vi "Test Type Check L2.vi"() -> ()   [LabVIEW 2021]
uses:
  ChannelCommon/typedef/FIFO Config.ctl
  ChannelCommon/ChannelCommon.lvlib
  CIFChannels/Typedef/Direction.ctl
  CIFChannels/CIFChannels.lvclass
  ChannelCommon/typedef/TimeStamps.ctl
  CIF_CIPC_L2Enet.lvclass
  FIFO_U8/CIF_CIPC_Fifo_U8.lvclass
  FIFO_Universal/CIF_CIPC_Universal.lvclass
panel:
  out "status":string
  out "pass":bool
  out "error out":errorcluster
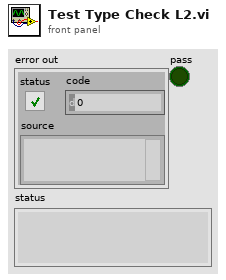
[diagram p1: front panel]
types:
  T1 = typedef "CIFChannels.lvclass/Direction.ctl" = enum16{"Publisher", "Subscriber"}
  T2 = typedef "ChannelCommon.lvlib/TimeStamps.ctl" = cluster{"ClockID":u8, "T0":i64, "T_Out":i64}
  T3 = typedef "ChannelCommon.lvlib/FIFO Config.ctl" = cluster{"Max Bytes/Msg":u64, "Max Msg/FIFO":u64, "Flags":u64}
  T4 = typedef "ChannelCommon.lvlib/New FIFO Instance Response.ctl" = cluster{"Publisher":string, "Custom Data":u8[]}
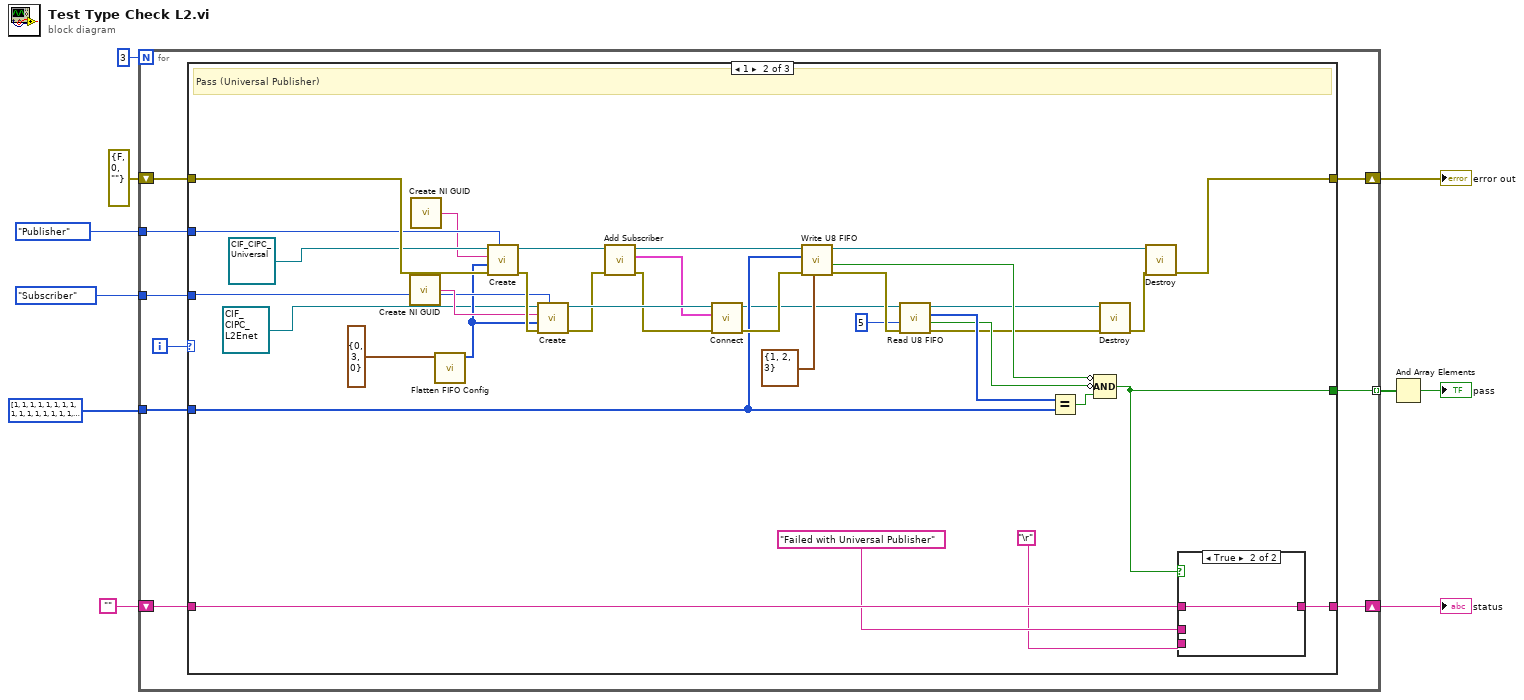
[diagram p0: block diagram]
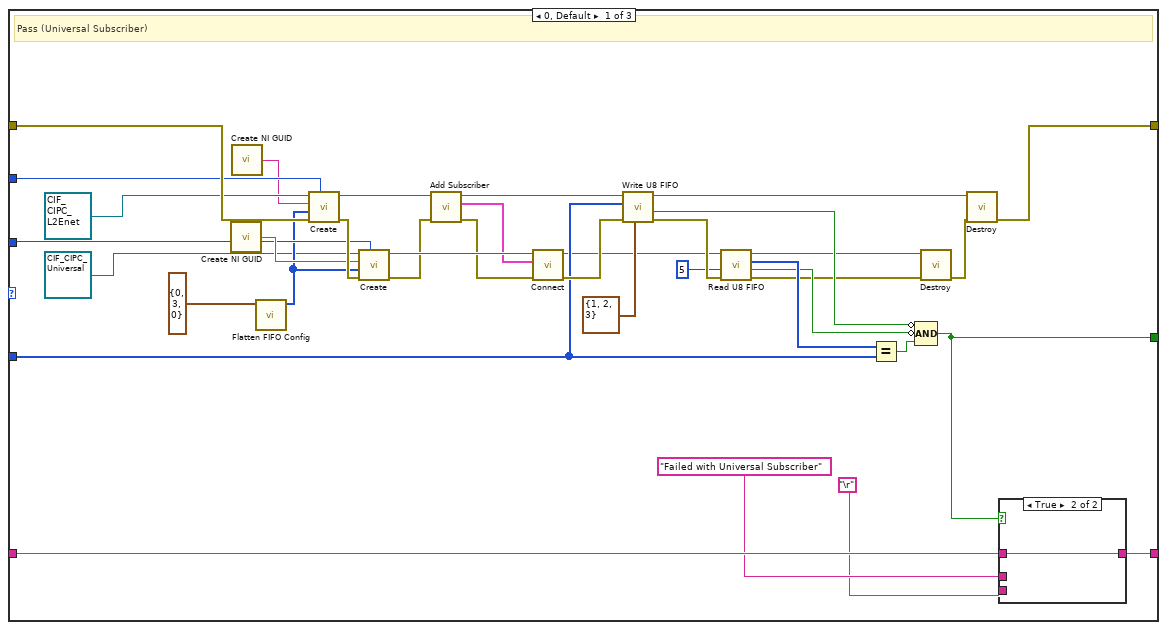
[diagram p2: hidden frame]
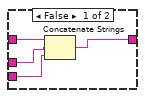
[diagram p3: hidden frame]
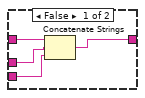
[diagram p4: hidden frame]
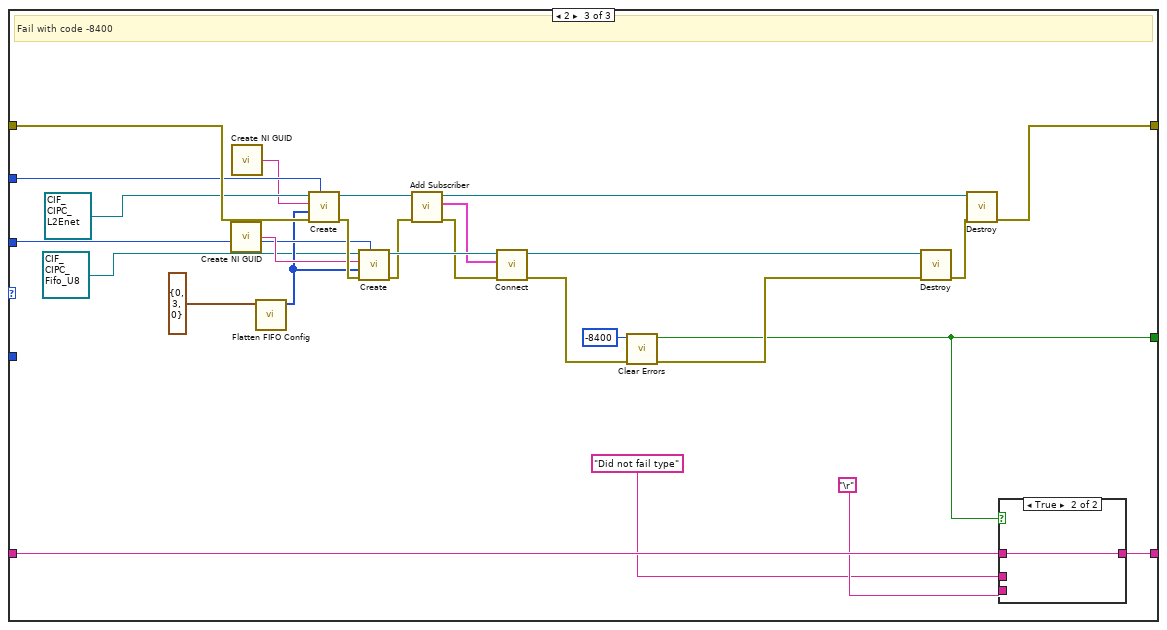
[diagram p5: hidden frame]
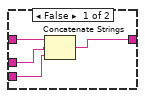
[diagram p6: hidden frame]
diagram:
  n1 = for {
    N: 3 -> [_]
    tunnel: [w19] -> w10 mode=indexing
    shift-right: [w12] -> w1
    shift-left: errorcluster {"status"=FALSE, "code"=0, "source"=""} ("error out") -> [w18]
    shift-right: [w15] -> w6
    shift-left: "" -> [w16]
    tunnel: Direction."Subscriber" ("Direction") -> [w14]
    tunnel: Direction."Publisher" ("Direction") -> [w13]
    tunnel: u8[] [1, 1, 1, 1, 1, 1, 1, 1, 1, 1, 1, 1, 1, 1, 1, 1, 1, 1, 1, 1, 1, 1, 1, 1, 1, 1, 1, 1, 1, 1, 1, 1, 1, 1, 1, 1, 1, 1, 1, 1, 1, 1, 1, 1, 1, 1, 1, 1, 1, 1, 1, 1, 1, 1, 1, 1, 1, 1, 1, 1, 1, 1, 1, 1, 1, 1, 1, 1, 1, 1, 1, 1, 1, 1, 1, 1, 1, 1, 1, 1, 1, 1, 1, 1, 1, 1, 1, 1, 1, 1, 1, 1, 1, 1, 1, 1, 1, 1, 1, 1, 1, 1, 1, 1, 1, 1, 1, 1, 1, 1, 1, 1, 1, 1, 1, 1, 1, 1, 1, 1, 1, 1, 1, 1, 1, 1, 1, 1, 1, 1, 1, 1, 1, 1, 1, 1, 1, 1, 1, 1, 1, 1, 1, 1, 1, 1, 1, 1, 1, 1, 1, 1, 1, 1, 1, 1, 1, 1, 1, 1, 1, 1, 1, 1, 1, 1, 1, 1, 1, 1, 1, 1, 1, 1, 1, 1, 1, 1, 1, 1, 1, 1, 1, 1, 1, 1, 1, 1, 1, 1, 1, 1, 1, 1, 1, 1, 1, 1, 1, 1, 1, 1, 1, 1, 1, 1, 1, 1, 1, 1, 1, 1, 1, 1, 1, 1, 1, 1, 1, 1, 1, 1, 1, 1, 1, 1, 1, 1, 1, 1, 1, 1, 1, 1, 1, 1, 1, 1, 1, 1, 1, 1, 1, 1, 1, 1, 1, 1, 1, 1, 1, 1, 1, 1, 1, 1, 1, 1, 1, 1, 1, 1, 1, 1, 1, 1, 1, 1, 1, 1, 1, 1, 1, 1, 1, 1, 1, 1, 1, 1, 1, 1, 1, 1, 1, 1, 1, 1, 1, 1, 1, 1, 1, 1, 1, 1, 1, 1, 1, 1, 1, 1, 1, 1, 1, 1, 1, 1, 1, 1, 1, 1, 1, 1, 1, 1, 1, 1, 1, 1, 1, 1, 1, 1, 1, 1, 1, 1, 1, 1, 1, 1, 1, 1, 1, 1, 1, 1, 1, 1, 1, 1, 1, 1, 1, 1, 1, 1, 1, 1, 1, 1, 1, 1, 1, 1, 1, 1, 1, 1, 1, 1, 1, 1, 1, 1, 1, 1, 1, 1, 1, 1, 1, 1, 1, 1, 1, 1, 1, 1, 1, 1, 1, 1, 1, 1, 1, 1, 1, 1, 1, 1, 1, 1, 1, 1, 1, 1, 1, 1, 1, 1, 1, 1, 1, 1, 1, 1, 1, 1, 1, 1, 1, 1, 1, 1, 1, 1, 1, 1, 1, 1, 1, 1, 1, 1, 1, 1, 1, 1, 1, 1, 1, 1, 1, 1, 1, 1, 1, 1, 1, 1, 1, 1, 1, 1, 1, 1, 1, 1, 1, 1, 1, 1, 1, 1, 1, 1, 1, 1, 1, 1, 1, 1, 1, 1, 1, 1, 1, 1, 1, 1, 1, 1, 1, 1, 1, 1, 1, 1, 1, 1, 1, 1, 1, 1, 1, 1, 1, 1, 1, 1, 1, 1, 1, 1, 1, 1, 1, 1, 1, 1, 1, 1, 1, 1, 1, 1, 1, 1, 1, 1, 1, 1, 1, 1, 1, 1, 1, 1, 1, 1, 1, 1, 1, 1, 1, 1, 1, 1, 1, 1, 1, 1, 1, 1, 1, 1, 1, 1, 1, 1, 1, 1, 1, 1, 1, 1, 1, 1, 1, 1, 1, 1, 1, 1, 1, 1, 1, 1, 1, 1, 1, 1, 1, 1, 1, 1, 1, 1, 1, 1, 1, 1, 1, 1, 1, 1, 1, 1, 1, 1, 1, 1, 1, 1, 1, 1, 1, 1, 1, 1, 1, 1, 1, 1, 1, 1, 1, 1, 1, 1, 1, 1, 1, 1, 1, 1, 1, 1, 1, 1, 1, 1, 1, 1, 1, 1, 1, 1, 1, 1, 1, 1, 1, 1, 1, 1, 1, 1, 1, 1, 1, 1, 1, 1, 1, 1, 1, 1, 1, 1, 1, 1, 1, 1, 1, 1, 1, 1, 1, 1, 1, 1, 1, 1, 1, 1, 1, 1, 1, 1, 1, 1, 1, 1, 1, 1, 1, 1, 1, 1, 1, 1, 1, 1, 1, 1, 1, 1, 1, 1, 1, 1, 1, 1, 1, 1, 1, 1, 1, 1, 1, 1, 1, 1, 1, 1, 1, 1, 1, 1, 1, 1, 1, 1, 1, 1, 1, 1, 1, 1, 1, 1, 1, 1, 1, 1, 1, 1, 1, 1, 1, 1, 1, 1, 1, 1, 1, 1, 1, 1, 1, 1, 1, 1, 1, 1, 1, 1, 1, 1, 1, 1, 1, 1, 1, 1, 1, 1, 1, 1, 1, 1, 1, 1, 1, 1, 1, 1, 1, 1, 1, 1, 1, 1, 1, 1, 1, 1, 1, 1, 1, 1, 1, 1, 1, 1, 1, 1, 1, 1, 1, 1, 1, 1, 1, 1, 1, 1, 1, 1, 1, 1, 1, 1, 1, 1, 1, 1, 1, 1, 1, 1, 1, 1, 1, 1, 1, 1, 1, 1, 1, 1, 1, 1, 1, 1, 1, 1, 1, 1, 1, 1, 1, 1, 1, 1, 1, 1, 1, 1, 1, 1, 1, 1, 1, 1, 1, 1, 1, 1, 1, 1, 1, 1, 1, 1, 1, 1, 1, 1, 1, 1, 1, 1, 1, 1, 1, 1, 1, 1, 1, 1, 1, 1, 1, 1, 1, 1, 1, 1, 1, 1, 1, 1, 1, 1, 1, 1, 1, 1, 1, 1, 1, 1, 1, 1, 1, 1, 1, 1, 1, 1, 1, 1, 1, 1, 1, 1, 1, 1, 1, 1, 1, 1, 1, 1, 1, 1, 1, 1, 1, 1, 1, 1, 1, 1, 1, 1, 1, 1, 1, 1, 1, 1, 1, 1, 1, 1, 1, 1, 1, 1, 1, 1, 1, 1, 1, 1, 1, 1, 1, 1, 1, 1, 1, 1, 1, 1, 1, 1, 1, 1, 1, 1, 1, 1, 1, 1, 1, 1, 1, 1, 1, 1, 1, 1, 1, 1, 1, 1, 1, 1, 1, 1, 1, 1, 1, 1, 1, 1, 1, 1, 1, 1, 1, 1, 1, 1, 1, 1, 1, 1, 1, 1, 1, 1, 1, 1, 1, 1, 1, 1, 1, 1, 1, 1, 1, 1, 1, 1, 1, 1, 1, 1, 1, 1, 1, 1, 1, 1, 1, 1, 1, 1, 1, 1, 1, 1, 1, 1, 1, 1, 1, 1, 1, 1, 1, 1, 1, 1, 1, 1, 1, 1, 1, 1, 1, 1, 1, 1, 1, 1, 1, 1, 1, 1, 1, 1, 1, 1, 1, 1, 1, 1, 1, 1, 1, 1, 1, 1, 1, 1, 1, 1, 1, 1, 1, 1, 1, 1, 1, 1, 1, 1, 1, 1, 1, 1, 1, 1, 1, 1, 1, 1, 1, 1, 1, 1, 1, 1, 1, 1, 1, 1, 1, 1, 1, 1, 1, 1, 1, 1, 1, 1, 1, 1, 1, 1, 1, 1, 1, 1, 1, 1, 1, 1, 1, 1, 1, 1, 1, 1, 1, 1, 1, 1, 1, 1, 1, 1, 1, 1, 1, 1, 1, 1, 1, 1, 1, 1, 1, 1, 1, 1, 1, 1, 1, 1, 1, 1, 1, 1, 1, 1, 1, 1, 1, 1, 1, 1, 1, 1, 1, 1, 1, 1, 1, 1, 1, 1, 1, 1, 1, 1, 1, 1, 1, 1, 1, 1, 1, 1, 1, 1, 1, 1, 1, 1, 1] ("Data in") -> [w11]
    i -> [w17]
    n2 = case shown="1" w17 {
      tunnel: [w50 w91 w108] -> w19
      tunnel: w18 -> [w48 w89 w124]
      tunnel: [w29 w71 w115] -> w12
      tunnel: w16 -> [w55 w96 w128]
      tunnel: [w54 w95 w127] -> w15
      tunnel: w14 -> [w46 w87 w122]
      tunnel: w13 -> [w45 w86 w121]
      tunnel: w11 -> [w34 w75 _]
      frame 0, Default {
        # "Pass (Universal Subscriber)"
        n3 = call <vilib>:"Create NI GUID.vi"() -> ("NI GUID"=w47:string)
        n4 = call <vilib>:"Create NI GUID.vi"() -> ("NI GUID"=w23:string)
        n5 = call "Flatten FIFO Config.vi"("FIFO Config in"=T3 {"Max Bytes/Msg"=0, "Max Msg/FIFO"=3, "Flags"=0}) -> ("Flattened FIFO Config"=w42:u8[])  [unwired: 10 in]
        n6 = call-dynamic "Create.vi"("Direction"=w45, "error in (no error)"=w48, "Custom Config Data"=w42, "Name"=w23, "CIFFIFO in"=refnum<class "CIF_CIPC_L2Enet.lvclass"> refnum ("CIF_DAQ_DVR_Multi.lvclass")) -> ("error out"=w49:errorcluster, "CIFFIFO out"=w25:refnum<class "CIF_CIPC_L2Enet.lvclass">)  [unwired: 5 in]
        n7 = call-dynamic "Create.vi"("Direction"=w46, "error in (no error)"=w49, "Custom Config Data"=w42, "Name"=w47, "CIFFIFO in"=refnum<class "CIF_CIPC_Universal.lvclass"> refnum ("CIF_CIPC_Universal.lvclass")) -> ("error out"=w21:errorcluster, "CIFFIFO out"=w43:refnum<class "CIF_CIPC_Universal.lvclass">)  [unwired: 5 in]
        n8 = call-dynamic "Add Subscriber.vi"("error in (no error)"=w21, "CIF_CIPC_Chn in"=w25) -> ("error out"=w20:errorcluster, "New FIFO Instance"=w22:T4, "CIF_CIPC_Chn out"=w24:refnum<class "CIF_CIPC_L2Enet.lvclass">)  [unwired: 7 in]
        n9 = call-dynamic "Connect.vi"("error in (no error)"=w20, "Connection"=w22, "CIFTag in"=w43) -> ("error out"=w41:errorcluster, "CIFTag out"=w28:refnum<class "CIF_CIPC_Universal.lvclass">)  [unwired: 7 in]
        n10 = call-dynamic "Write U8 FIFO.vi"("FIFO Timestamps"=T2 {"ClockID"=1, "T0"=2, "T_Out"=3}, "error in (no error)"=w41, "Data in"=w34, "CIFFIFO in"=w24) -> ("error out"=w37:errorcluster, "timed out?"=w40:bool, "CIFFIFO out"=w27:refnum<class "CIF_CIPC_L2Enet.lvclass">)  [unwired: 4 in, 1 out]
        n11 = call-dynamic "Read U8 FIFO.vi"("error in (no error)"=w37, "Timeout (ms)"=5, "CIFFIFO in"=w28) -> ("error out"=w31:errorcluster, "timed out?"=w38:bool, "Data out"=w39:u8[], "CIFFIFO out"=w32:refnum<class "CIF_CIPC_Universal.lvclass">)  [unwired: 4 in, 1 out]
        n12 = Equal?(x=w39, y=w34) -> (x = y?=w51:bool)
        n13 = Compound Arithmetic op=AND(invert w40, invert w38, w51) -> (w50:bool)
        n14 = call-dynamic "Destroy.vi"("error in (no error)"=w31, "CIFTag in"=w32) -> ("error out"=w30:errorcluster)  [unwired: 8 in, 1 out]
        n15 = call-dynamic "Destroy.vi"("error in (no error)"=w30, "CIFTag in"=w27) -> ("error out"=w29:errorcluster)  [unwired: 8 in, 1 out]
        n16 = case shown="True" w50 {
          tunnel: w55 -> [w59 w60]
          tunnel: [w56 w60] -> w54
          tunnel: "Failed with Universal Subscriber" -> [w58 _]
          tunnel: "\r" -> [w57 _]
          frame False {
            n17 = Concatenate Strings(w59, w58, w57) -> (w56:string)
          }
          frame True {
          }
        }
      }
      frame 1 {
        # "Pass (Universal Publisher)"
        n18 = call <vilib>:"Create NI GUID.vi"() -> ("NI GUID"=w88:string)
        n19 = call <vilib>:"Create NI GUID.vi"() -> ("NI GUID"=w63:string)
        n20 = call "Flatten FIFO Config.vi"("FIFO Config in"=T3 {"Max Bytes/Msg"=0, "Max Msg/FIFO"=3, "Flags"=0}) -> ("Flattened FIFO Config"=w83:u8[])  [unwired: 10 in]
        n21 = call-dynamic "Create.vi"("Direction"=w86, "error in (no error)"=w89, "Custom Config Data"=w83, "Name"=w63, "CIFFIFO in"=refnum<class "CIF_CIPC_Universal.lvclass"> refnum ("CIF_CIPC_Universal.lvclass")) -> ("error out"=w90:errorcluster, "CIFFIFO out"=w66:refnum<class "CIF_CIPC_Universal.lvclass">)  [unwired: 5 in]
        n22 = call-dynamic "Create.vi"("Direction"=w87, "error in (no error)"=w90, "Custom Config Data"=w83, "Name"=w88, "CIFFIFO in"=refnum<class "CIF_CIPC_L2Enet.lvclass"> refnum ("CIF_DAQ_DVR_Multi.lvclass")) -> ("error out"=w65:errorcluster, "CIFFIFO out"=w84:refnum<class "CIF_CIPC_L2Enet.lvclass">)  [unwired: 5 in]
        n23 = call-dynamic "Add Subscriber.vi"("error in (no error)"=w65, "CIF_CIPC_Chn in"=w66) -> ("error out"=w64:errorcluster, "New FIFO Instance"=w62:T4, "CIF_CIPC_Chn out"=w61:refnum<class "CIF_CIPC_Universal.lvclass">)  [unwired: 7 in]
        n24 = call-dynamic "Connect.vi"("error in (no error)"=w64, "Connection"=w62, "CIFTag in"=w84) -> ("error out"=w82:errorcluster, "CIFTag out"=w70:refnum<class "CIF_CIPC_L2Enet.lvclass">)  [unwired: 7 in]
        n25 = call-dynamic "Write U8 FIFO.vi"("FIFO Timestamps"=T2 {"ClockID"=1, "T0"=2, "T_Out"=3}, "error in (no error)"=w82, "Data in"=w75, "CIFFIFO in"=w61) -> ("error out"=w78:errorcluster, "timed out?"=w81:bool, "CIFFIFO out"=w69:refnum<class "CIF_CIPC_Universal.lvclass">)  [unwired: 4 in, 1 out]
        n26 = call-dynamic "Read U8 FIFO.vi"("error in (no error)"=w78, "Timeout (ms)"=5, "CIFFIFO in"=w70) -> ("error out"=w73:errorcluster, "timed out?"=w79:bool, "Data out"=w80:u8[], "CIFFIFO out"=w74:refnum<class "CIF_CIPC_L2Enet.lvclass">)  [unwired: 4 in, 1 out]
        n27 = Equal?(x=w80, y=w75) -> (x = y?=w92:bool)
        n28 = Compound Arithmetic op=AND(invert w81, invert w79, w92) -> (w91:bool)
        n29 = call-dynamic "Destroy.vi"("error in (no error)"=w73, "CIFTag in"=w74) -> ("error out"=w72:errorcluster)  [unwired: 8 in, 1 out]
        n30 = call-dynamic "Destroy.vi"("error in (no error)"=w72, "CIFTag in"=w69) -> ("error out"=w71:errorcluster)  [unwired: 8 in, 1 out]
        n31 = case shown="True" w91 {
          tunnel: w96 -> [w100 w101]
          tunnel: [w97 w101] -> w95
          tunnel: "Failed with Universal Publisher" -> [w99 _]
          tunnel: "\r" -> [w98 _]
          frame False {
            n32 = Concatenate Strings(w100, w99, w98) -> (w97:string)
          }
          frame True {
          }
        }
      }
      frame 2 {
        # "Fail with code -8400"
        n33 = call <vilib>:"Create NI GUID.vi"() -> ("NI GUID"=w123:string)
        n34 = call <vilib>:"Create NI GUID.vi"() -> ("NI GUID"=w103:string)
        n35 = call "Flatten FIFO Config.vi"("FIFO Config in"=T3 {"Max Bytes/Msg"=0, "Max Msg/FIFO"=3, "Flags"=0}) -> ("Flattened FIFO Config"=w118:u8[])  [unwired: 10 in]
        n36 = call-dynamic "Create.vi"("Direction"=w121, "error in (no error)"=w124, "Custom Config Data"=w118, "Name"=w103, "CIFFIFO in"=refnum<class "CIF_CIPC_L2Enet.lvclass"> refnum ("CIF_DAQ_DVR_Multi.lvclass")) -> ("error out"=w125:errorcluster, "CIFFIFO out"=w107:refnum<class "CIF_CIPC_L2Enet.lvclass">)  [unwired: 5 in]
        n37 = call-dynamic "Create.vi"("Direction"=w122, "error in (no error)"=w125, "Custom Config Data"=w118, "Name"=w123, "CIFFIFO in"=refnum<class "CIF_CIPC_Fifo_U8.lvclass"> refnum ("CIF_CIPC_Fifo_U8.lvclass")) -> ("error out"=w106:errorcluster, "CIFFIFO out"=w119:refnum<class "CIF_CIPC_Fifo_U8.lvclass">)  [unwired: 5 in]
        n38 = call-dynamic "Add Subscriber.vi"("error in (no error)"=w106, "CIF_CIPC_Chn in"=w107) -> ("error out"=w105:errorcluster, "New FIFO Instance"=w102:T4, "CIF_CIPC_Chn out"=w104:refnum<class "CIF_CIPC_L2Enet.lvclass">)  [unwired: 7 in]
        n39 = call-dynamic "Connect.vi"("error in (no error)"=w105, "Connection"=w102, "CIFTag in"=w119) -> ("error out"=w112:errorcluster, "CIFTag out"=w110:refnum<class "CIF_CIPC_Fifo_U8.lvclass">)  [unwired: 7 in]
        n40 = call <vilib>:"Clear Errors.vi"("error in (no error)"=w112, "specific error code to clear (0: all)"=-8400) -> ("error out"=w109:errorcluster, "specific error cleared?"=w108:bool)  [unwired: 4 in]
        n41 = call-dynamic "Destroy.vi"("error in (no error)"=w109, "CIFTag in"=w110) -> ("error out"=w116:errorcluster)  [unwired: 8 in, 1 out]
        n42 = call-dynamic "Destroy.vi"("error in (no error)"=w116, "CIFTag in"=w104) -> ("error out"=w115:errorcluster)  [unwired: 8 in, 1 out]
        n43 = case shown="True" w108 {
          tunnel: w128 -> [w132 w133]
          tunnel: [w129 w133] -> w127
          tunnel: "Did not fail type" -> [w131 _]
          tunnel: "\r" -> [w130 _]
          frame False {
            n44 = Concatenate Strings(w132, w131, w130) -> (w129:string)
          }
          frame True {
          }
        }
      }
    }
  }
  "error out" <- w1
  "status" <- w6
  n45 = And Array Elements(Boolean array=w10) -> (logical AND=→"pass":bool)
